vi "例10.1  利用底层函数采集单幅图像.vi"() -> ()   [LabVIEW 2017]
doc: "The Snap VI acquires an image and displays the image in an image control using low-level acquisition VIs. A snap is appropriate for low-speed or single-capture applications in which ease of programming is essential."
uses:
  <vilib>/userdefined/High Color/IMAQdx.ctl
  <vilib>/vision/driver/IMAQdx.llb/IMAQdx Acquisition Mode.ctl
  <vilib>/vision/driver/IMAQdx.llb/IMAQdx Buffer Number Mode.ctl
  <vilib>/vision/driver/NI_Vision_Acquisition_Software.lvlib
panel:
  in  "Camera Name":T1
  out "Image":T2(plugin-control)
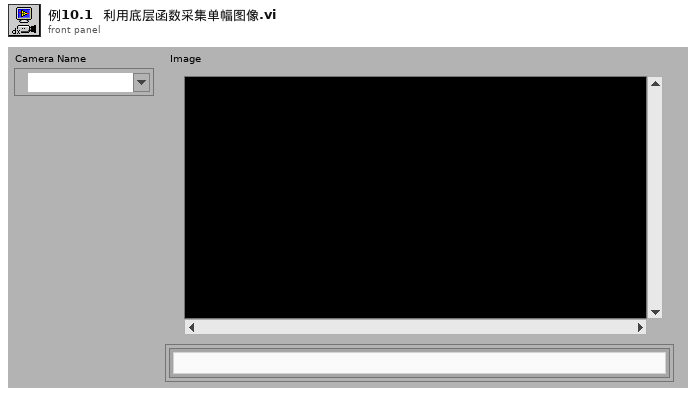
[diagram p1: front panel]
types:
  T1 = typedef "IMAQdx.ctl" = refnum<k21>
  T2 = typedef "IMAQ Image.ctl" = refnum<image>
  T3 = typedef "NI_Vision_Acquisition_Software.lvlib/IMAQdx Buffer Number Mode.ctl" = enum32{"Next", "Last", "Buffer Number", "Every", "Last New"}
  T4 = typedef "NI_Vision_Acquisition_Software.lvlib/IMAQdx Acquisition Mode.ctl" = enum32{"One Shot", "Continuous"}
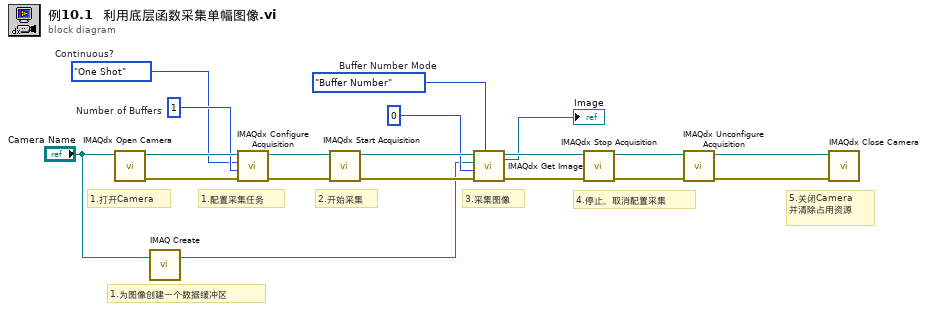
[diagram p0: block diagram]
diagram:
  w11 = IMAQdx_Buffer_Number_Mode."Buffer Number"  # Buffer Number Mode
  w12 = u32 1  # Number of Buffers
  w4 = IMAQdx_Acquisition_Mode."One Shot"  # Continuous?
  # "5.关闭Camera\n并清除占用资源"
  # "1.为图像创建一个数据缓冲区"
  # "4.停止、取消配置采集"
  # "3.采集图像"
  # "2.开始采集"
  # "1.配置采集任务"
  # "1.打开Camera"
  n1 = call <vilib>:"IMAQdx Open Camera.vi"("Session In"="Camera Name") -> ("error out"=w15:errorcluster, "Session Out"=w17:T1)  [unwired: 2 in, 7 out]
  n2 = call "IMAQ Create"("Image Name"="Camera Name") -> ("New Image"=w1:T2)  [unwired: 3 in, 2 out]
  n3 = call <vilib>:"IMAQdx Configure Acquisition.vi"("error in"=w15, "Number of Buffers"=w12, "Continuous?"=w4, "Session In"=w17) -> ("error out"=w18:errorcluster, "Session Out"=w16:T1)  [unwired: 6 out]
  n4 = call <vilib>:"IMAQdx Start Acquisition.vi"("error in"=w18, "Session In"=w16) -> ("error out"=w14:errorcluster, "Session Out"=w13:T1)  [unwired: 8 out]
  n5 = call <vilib>:"IMAQdx Get Image.vi"("Buffer Number Mode (Next)"=w11, "error in"=w14, "Buffer Number In"=u32 0, "Image In"=w1, "Session In"=w13) -> ("error out"=w3:errorcluster, "Image Out"=→"Image":T2, "Session Out"=w6:T1)  [unwired: 4 out]
  n6 = call <vilib>:"IMAQdx Stop Acquisition.vi"("error in"=w3, "Session In"=w6) -> ("error out"=w9:errorcluster, "Session Out"=w2:T1)  [unwired: 8 out]
  n7 = call <vilib>:"IMAQdx Unconfigure Acquisition.vi"("error in"=w9, "Session In"=w2) -> ("error out"=w8:errorcluster, "Session Out"=w7:T1)  [unwired: 8 out]
  n8 = call <vilib>:"IMAQdx Close Camera.vi"("error in"=w8, "Session In"=w7) -> ()  [unwired: 10 out]
